vi "Temperature Controller Main.vi"() -> ()   [LabVIEW 2019, in "Controller.lvlib"]
uses:
  Controller.lvlib
  source code/LSL components/scripts/scripts manager/scripts manager.lvclass
  source code/LSL components/output terminal/Plain OT/PainOutputTerminal.lvclass
  D:/Pet Projects/LSL/source code/LSL components/output terminal/Base/Output Terminal.lvclass
  source code/LSL components/output terminal/Plain OT/PainOutputTerminal.lvclass/PainOutputTerminal.ctl
  source code/LSL components/variables/RT Variables/RT Variables.lvclass
  source code/LSL components/scripts/scripts manager/scripts manager.lvclass/scripts manager.ctl
  source code/LSL components/output terminal/Plain OT/properties/Write Output Terminal.vi
  source code/LSL components/scripts/scripts manager/properties/Write Scripts.vi
  customfunctions/ControllerData/ControllerData.lvclass
panel:
  out "Heater State":bool
  in  "Low Limit":dbl
  in  "High Limit":dbl
  out "CurrentTemperature":dbl(slide) scale=0.0..100.0
  out "Heater State Trend":i16(graph)
  out "Temperature Trend":T1(graph)
  in  "Script Run":bool
  in  "Script Editor":string
  out "Output Terminal":string
  # "Temperature Controller running on windows"
  # "Debug Console"
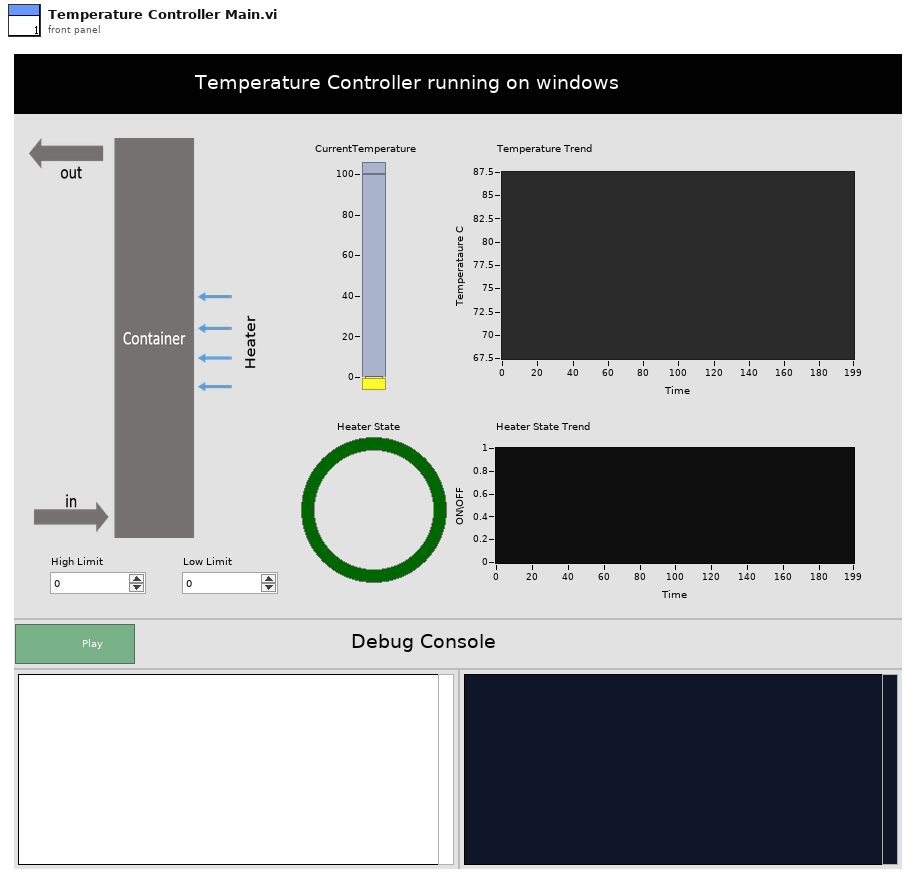
[diagram p1: front panel]
types:
  T1 = cluster{"Current Temp":dbl, "Low Set Point":dbl, "High Set Point":dbl}
  T2 = enum32{"invalid app kind", "Development System", "Run Time System", "Student Edition", "Embedded LabVIEW", "Evaluation", "Custom"}
  T3 = cluster{"Current Temp":dbl, "Low Set Point":dbl, "High Set Point":dbl}[]
  T4 = enum32{"Invalid", "Standard", "Closed", "Hidden", "Minimized", "Maximized"}
  T5 = cluster{"Core":cluster{"Current VI Reference":refnum<vi>, "Close Panel on Exit?":bool}, "High Set Point":dbl, "Low Set Point":dbl, "Current Temp":dbl, "Heater ON?":bool, "scripts manager":refnum<class "scripts manager.lvclass">, "Terminal":refnum<class "PainOutputTerminal.lvclass">, "appended path":path}
  T6 = cluster{"Current VI Reference":refnum<vi>, "Close Panel on Exit?":bool}
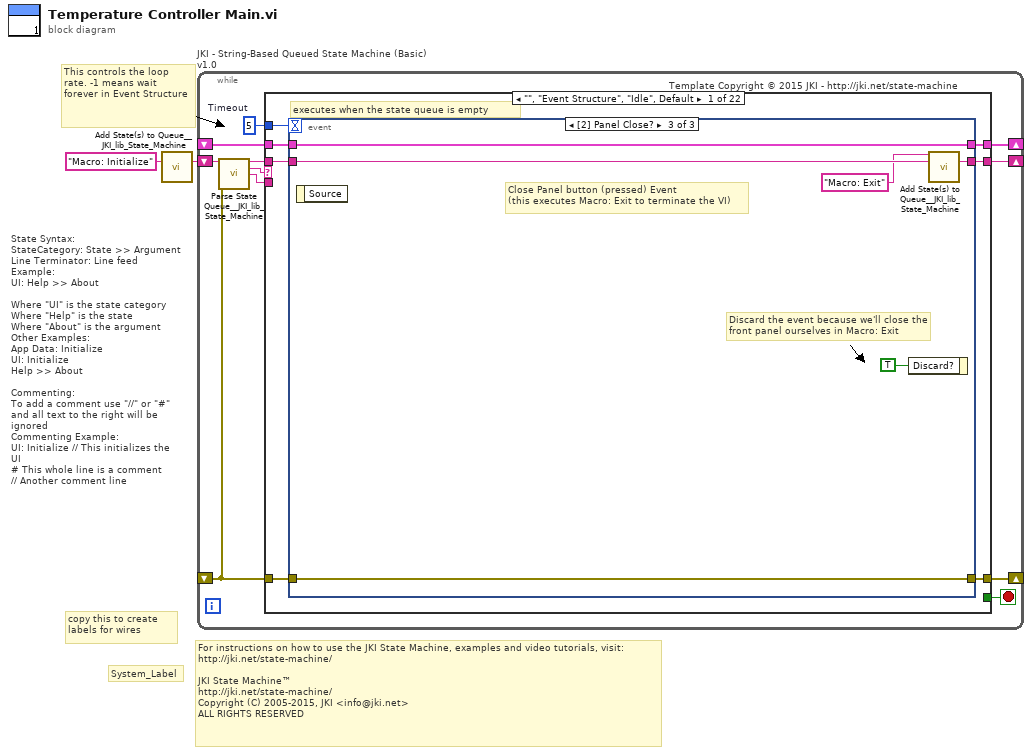
[diagram p0: block diagram]
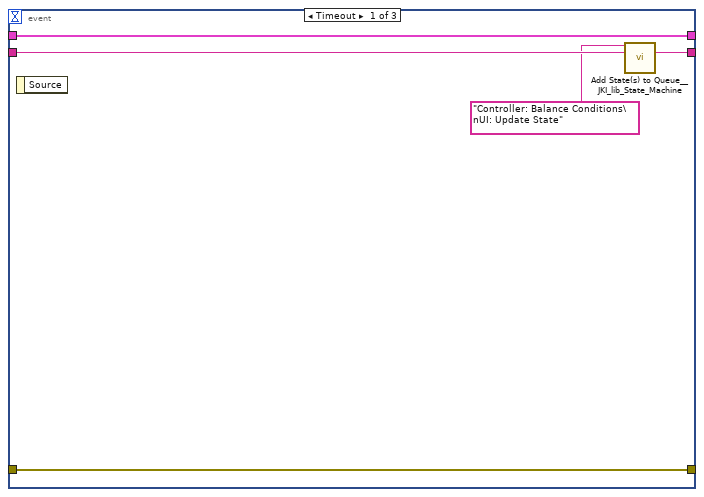
[diagram p2: hidden frame]
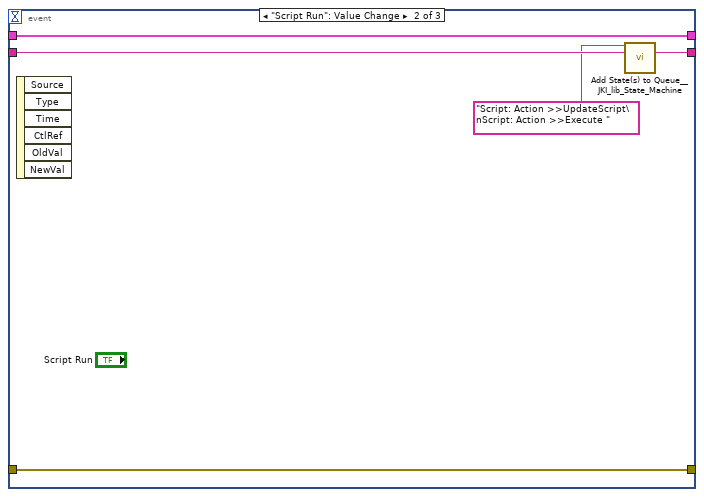
[diagram p3: hidden frame]
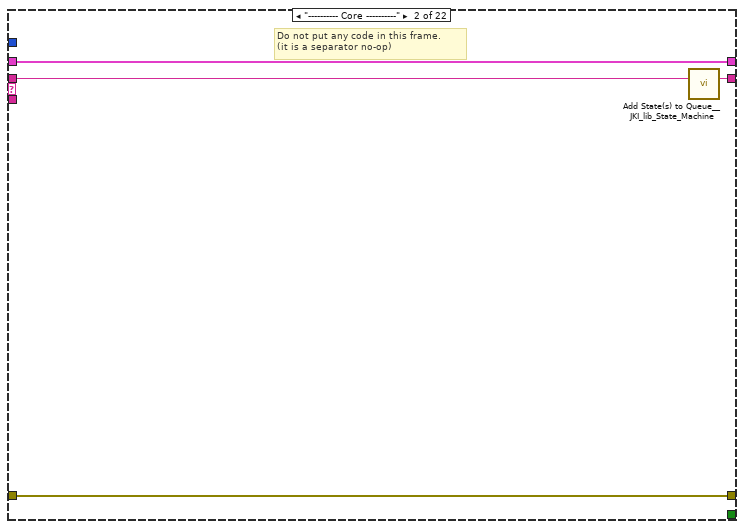
[diagram p4: hidden frame]
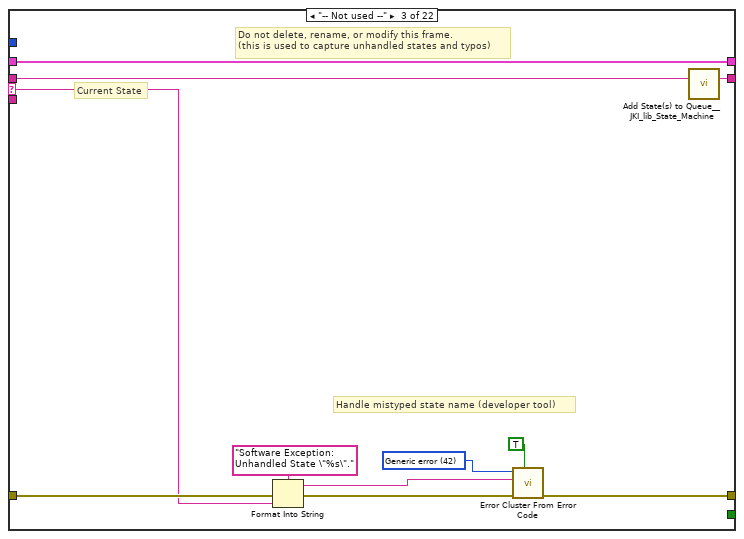
[diagram p5: hidden frame]
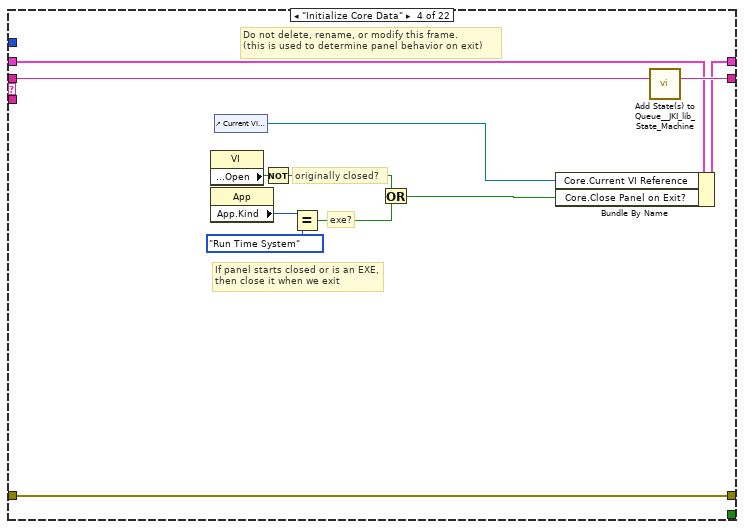
[diagram p6: hidden frame]
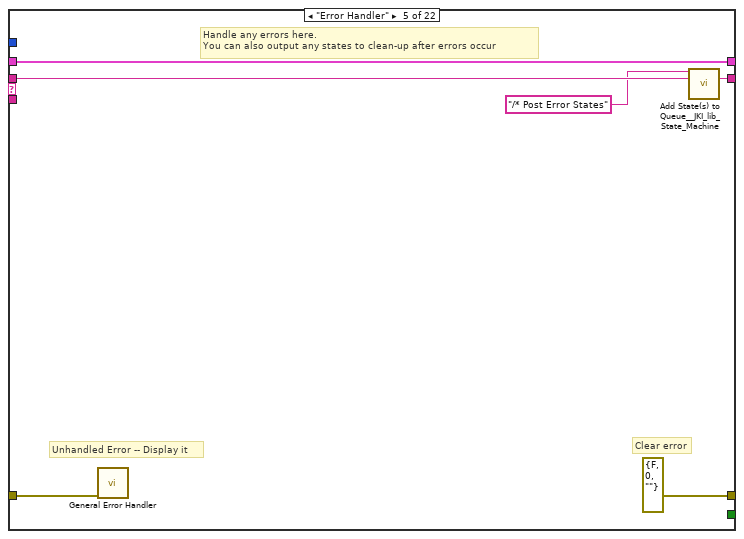
[diagram p7: hidden frame]
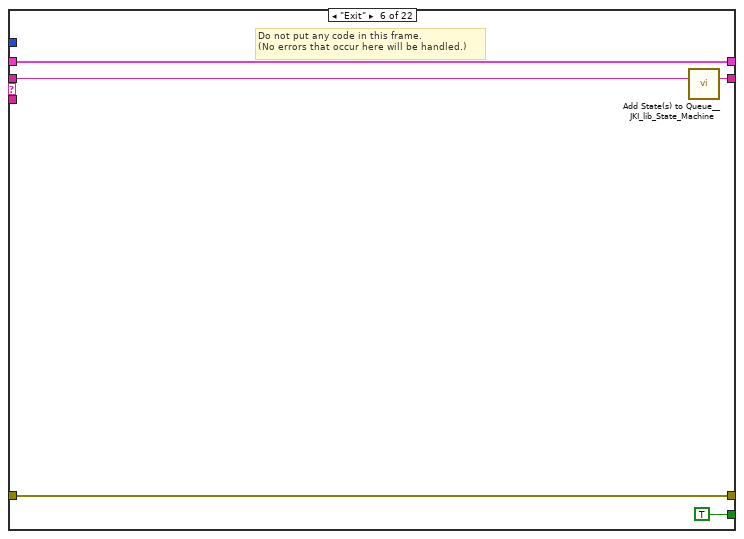
[diagram p8: hidden frame]
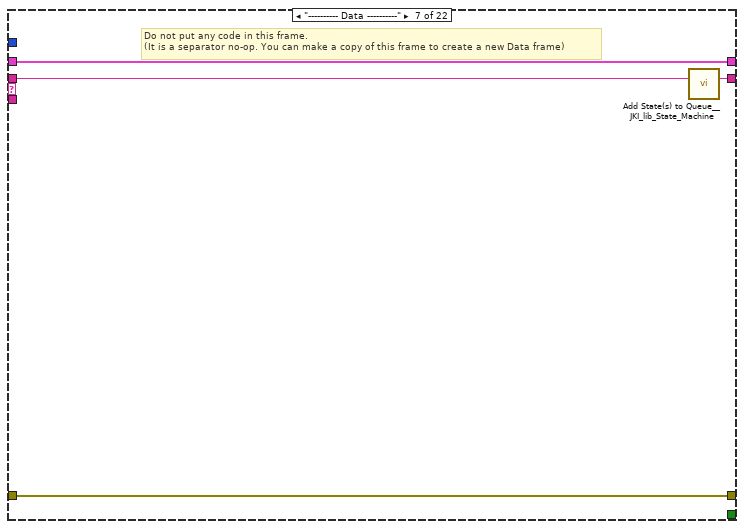
[diagram p9: hidden frame]
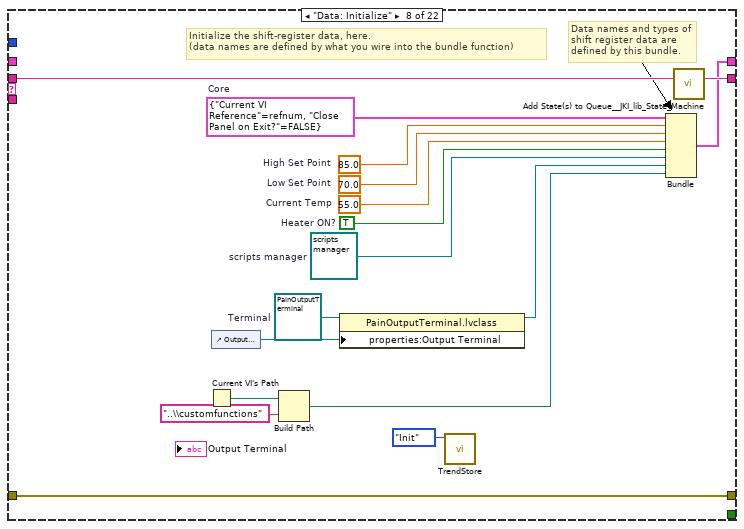
[diagram p10: hidden frame]
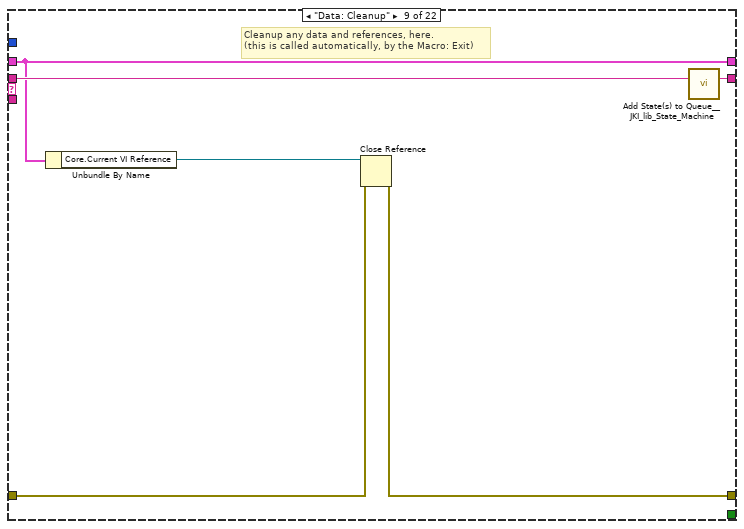
[diagram p11: hidden frame]
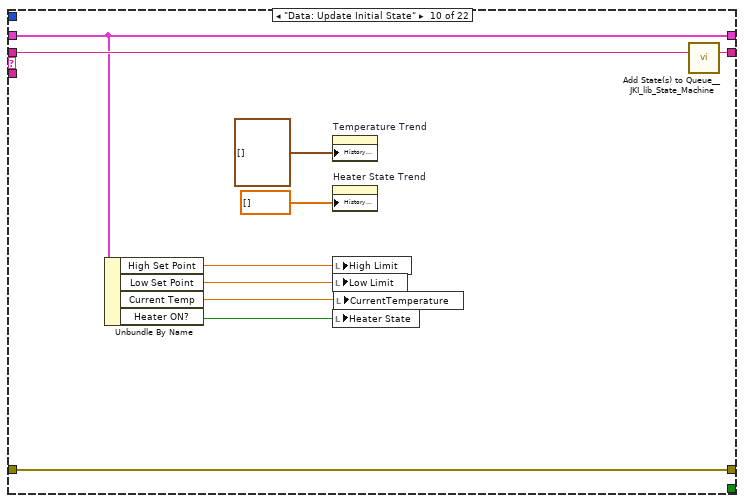
[diagram p12: hidden frame]
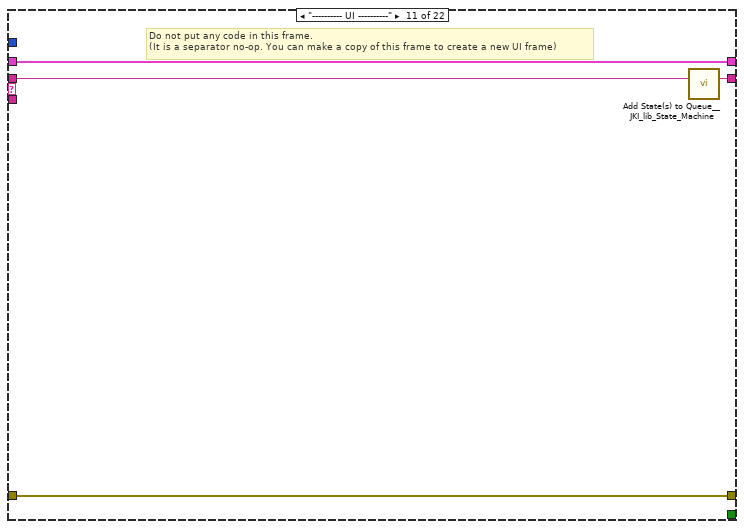
[diagram p13: hidden frame]
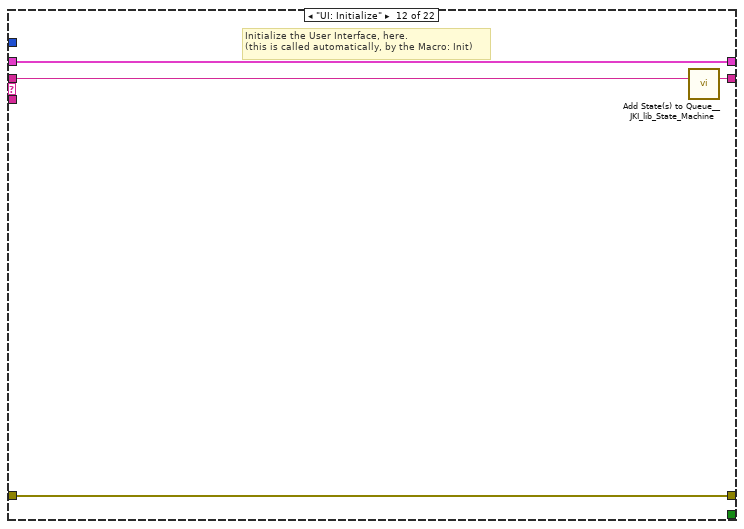
[diagram p14: hidden frame]
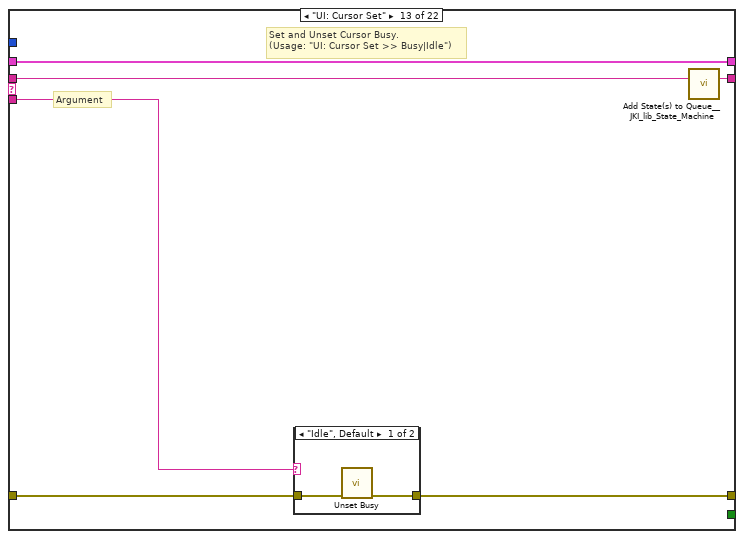
[diagram p15: hidden frame]
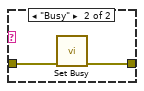
[diagram p16: hidden frame]
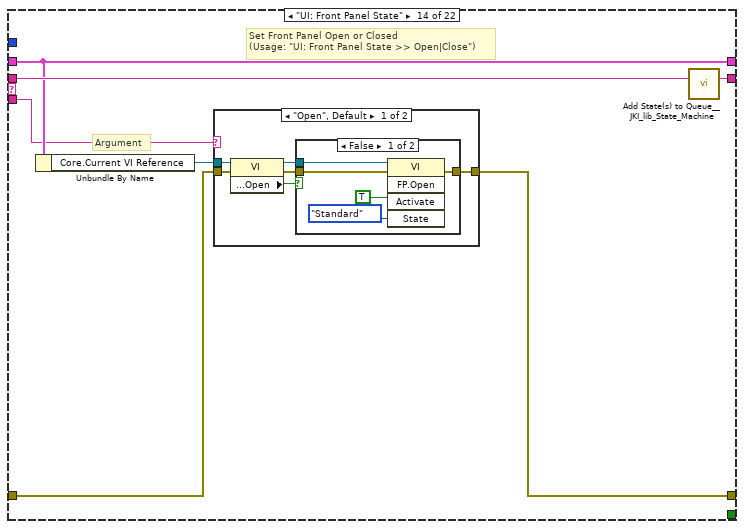
[diagram p17: hidden frame]
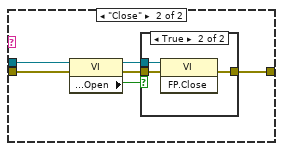
[diagram p19: hidden frame]
diagram:
  # "For instructions on how to use the JKI State Machine, examples and video tutorials, visit:\nhttp://jki.net/state-machine/\n\nJKI State Machine™\nhttp://jki.net/state-machine/\nCopyright (C) 2005-2015, JKI <info@jki.net>\nALL RIGHTS RESERVED"
  # "State Syntax:\nStateCategory: State >> Argument\nLine Terminator: Line feed\nExample:\nUI: Help >> About\n\nWhere \"UI\" is the state category\nWhere \"Help\" is the state\nWhere \"About\" is the argument\nOther Examples:\nApp Data: Initialize\nUI: Initialize\nHelp >> About\n\nCommenting:\nTo add a comment use \"//\" or \"#\" and all text to the right will be ignored\nCommenting Example:\nUI: Initialize // This initializes the UI\n# This whole line is a comment\n// Another comment line"
  # "copy this to create labels for wires"
  # "This controls the loop rate. -1 means wait forever in Event Structure"
  # "System_Label"
  n1 = call <vilib>:"Add State(s) to Queue__JKI_lib_State_Machine.vi"("State(s) in (\"\")"="Macro: Initialize") -> ("States Out"=w2:string)  [unwired: 14 in]
  n2 = while "JKI - String-Based Queued State Machine (Basic) v1.0" {
    shift-right: [w6] -> _
    shift-left: _ -> [w5]
    shift-right: [w9] -> _
    shift-left: _ -> [w3]
    shift-right: [w8] -> _
    shift-left: w2 -> [w10]
    stop <- w7 stop-if-true
    w4 = 5  # Timeout
    # "Template Copyright © 2015 JKI - http://jki.net/state-machine"
    n3 = call <vilib>:"Parse State Queue__JKI_lib_State_Machine.vi"("State Queue"=w10, "Error In (no error)"=w3) -> ("Remaining States"=w12:string, "Current State"=w13:string, "Arguments"=w11:string)  [unwired: 11 in]
    n4 = case shown="\"\", \"Event Structure\", \"Idle\", Default" w13 {
      selector: w13 -> [_ _ w41 _ _ _ _ _ _ _ _ _ _ _ _ _ _ _ _ _ _ _]
      tunnel: w12 -> [w20 w40 w45 w63 w69 w74 w78 w95 w101 w111 w115 w119 w125 w136 w167 w172 w177 w187 w191 w210 w212 w223]
      tunnel: w11 -> [_ _ _ _ _ _ _ _ _ _ _ _ w120 w130 _ _ _ _ _ _ _ w222]
      tunnel: w5 -> [w18 w37 w43 w54 w66 w72 w75 _ w96 w106 w112 w117 w123 w132 w165 w169 w174 w184 w188 w205 w213 w218]
      tunnel: [w17 w38 w47 w60 errorcluster {"status"=FALSE, "code"=0, "source"=""} ("error out") w71 w76 w92 w97 w109 w113 w116 w121 w133 w168 w170 w175 w185 w189 w208 w211 w216] -> w9
      tunnel: w3 -> [w16 w38 w46 w60 w65 w71 w76 w92 w98 w109 w113 w116 w122 w134 w168 w170 w175 w185 w189 w208 w211 w217]
      tunnel: [w19 w39 w44 w62 w68 w73 w77 w94 w100 w110 w114 w118 w124 w135 w166 w171 w176 w186 w190 w209 w212 w223] -> w8
      tunnel: [_ _ _ _ _ TRUE _ _ _ _ _ _ _ _ _ _ _ _ _ _ _ _] -> w7
      tunnel: [w15 w37 w43 w61 w66 w72 w75 w93 w96 w106 w112 w117 w123 w132 w165 w169 w174 w184 w188 w204 w213 w219] -> w6
      tunnel: w4 -> [w14 _ _ _ _ _ _ _ _ _ _ _ _ _ _ _ _ _ _ _ _ _]
      frame "", "Event Structure", "Idle", Default {
        # "executes when the state queue is empty"
        n5 = event shown="[2] Panel Close?" {
          selector: _ -> [_ _ _]
          dyn-events: _ -> [_ _ _]
          timeout: w14 -> [_ _ _]
          tunnel: w20 -> [w25 w30 w36]
          tunnel: [w24 w29 w35] -> w19
          tunnel: w18 -> [w22 w27 w33]
          tunnel: [w23 w28 w34] -> w17
          tunnel: w16 -> [w23 w28 w34]
          tunnel: [w22 w27 w33] -> w15
          event Timeout {
            n6 = event-data() -> ()  [unwired: 1 in, 1 out]
            n7 = call <vilib>:"Add State(s) to Queue__JKI_lib_State_Machine.vi"("State(s) in Front (\"\")"="Controller: Balance Conditions\nUI: Update State" ("State(s) in Front (\"\")"), "State(s) in (\"\")"=w25) -> ("States Out"=w24:string)  [unwired: 13 in]
          }
          event "Script Run": Value Change {
            n8 = event-data() -> ()  [unwired: 1 in, 6 out]
            n9 = call <vilib>:"Add State(s) to Queue__JKI_lib_State_Machine.vi"("State(s) in Front (\"\")"="Script: Action >>UpdateScript\nScript: Action >>Execute " ("State(s) in Front (\"\")"), "State(s) in (\"\")"=w30) -> ("States Out"=w29:string)  [unwired: 13 in]
          }
          event Panel Close? {
            # "Discard the event because we'll close the front panel ourselves in Macro: Exit"
            # "Close Panel button (pressed) Event\n(this executes Macro: Exit to terminate the VI)"
            n10 = event-data() -> ()  [unwired: 1 in, 1 out]
            n11 = event-data("Discard?"=TRUE) -> ()  [unwired: 1 in, 1 out]
            n12 = call <vilib>:"Add State(s) to Queue__JKI_lib_State_Machine.vi"("State(s) in Front (\"\")"="Macro: Exit", "State(s) in (\"\")"=w36) -> ("States Out"=w35:string)  [unwired: 13 in]
          }
        }
      }
      frame "---------- Core ----------" {
        # "Do not put any code in this frame.\n(it is a separator no-op)"
        n13 = call <vilib>:"Add State(s) to Queue__JKI_lib_State_Machine.vi"("State(s) in (\"\")"=w40) -> ("States Out"=w39:string)  [unwired: 14 in]
      }
      frame "-- Not used --" {
        w50 = 42 items=["No error", "Argument error", "Memory is full", "Out of zone", "End of file", "File already open", "Generic file I/O error", "File not found", "File permission error", "Disk is full", "Duplicate path", "Too many files open", "System feature not enabled", "Resource file not found", "Cannot add resource", "Resource not found", "Image not found", "Image memory error", "Pen does not exist", "Config type invalid", "Config token not found", "Config parse error", "Config memory error", "Bad external code format", "Bad external code offset", "External code not present", "Null window", "Destroy window error", "Null menu", "Print aborted", "Bad print record", "Print driver error", "Windows error during printing", "Memory error during printing", "Print dialog error", "Generic print error", "Invalid device refnum", "Device not found", "Device parameter error", "Device unit error", "Cannot open device", "Device call aborted", "Generic error", "Cancelled by user", "Object ID too low", "Object ID too high", "Object not in heap", "Unknown heap", "Unknown object (invalid DefProc)", "Unknown object (DefProc not in table)", "Message out of range", "Invalid (null) method", "Unknown message", "Manager call not supported", "Bad address", "Network operation in progress", "Network operation timed out", "Connection is busy", "Network attribute not supported", "Network error", "Address in use", "System out of memory", "Connection aborted", "Connection refused", "Not connected", "Already connected", "Connection closed", "Initialization error (interapplication manager)", "Bad occurrence", "Wait on unbound occurrence handler", "Occurrence queue overflow", "Datalog type conflict", "Unused", "Unrecognized type (interapplication manager)", "Memory corrupt", "Failed to make temporary DLL", "Old CIN version", "Drag socket not found", "Failed to load drop-object", "Failed to register OLE object", "Failed to release OLE object", "Format specifier type mismatch", "Unknown format specifier", "Too few format specifiers", "Too many format specifiers", "Scan failed", "Newer CIN version", "Error converting to variant", "Runtime menu error", "Password tampered", "Variant attribute not found", "Incompatible variant data type", "Event data is not available", "Event Store is not present", "Occurrence is not found", "Event Queue is not created", "Event info is not available", "Refnum passed is NULL", "Error retrieving Class GUID", "Error retrieving CoClass GUID", "Error retrieving TypeLib GUID.", "Bad built application magic bytes.", "Specific driver is different from the specific driver associated with the Logical Name.", "There is no session opened to the class driver.", "Max Error", "MAX - Error with config objects", "MAX - Error loading configuration", "MAX - Group not supported"]
        # "Current State"
        # "Do not delete, rename, or modify this frame.\n(this is used to capture unhandled states and typos)"
        # "Handle mistyped state name (developer tool)"
        n14 = Format Into String(format string="Software Exception: Unhandled State \"%s\"." ("message"), error in=w46, w41) -> (resulting string=w49:string, error out=w48:errorcluster)  [unwired: 1 in]
        n15 = call <vilib>:"Error Cluster From Error Code.vi"("show call chain? (False)"=TRUE, "error in (no error)"=w48, "error message (\"\")"=w49, "error code (0)"=w50) -> ("error out"=w47:errorcluster)  [unwired: 5 in]
        n16 = call <vilib>:"Add State(s) to Queue__JKI_lib_State_Machine.vi"("State(s) in (\"\")"=w45) -> ("States Out"=w44:string)  [unwired: 14 in]
      }
      frame "Initialize Core Data" {
        # "Do not delete, rename, or modify this frame.\n(this is used to determine panel behavior on exit)"
        # "originally closed?"
        # "exe?"
        # "If panel starts closed or is an EXE, then close it when we exit"
        n17 = property class="VI"() -> ("Front Panel.Open"=w59:bool)  [unwired: 2 in, 2 out]
        n18 = property class="App"() -> ("App.Kind"=w58:T2)  [unwired: 2 in, 2 out]
        n19 = control-ref of="Current VI Reference"() -> (w52:refnum<vi>)
        n20 = Not(x=w59) -> (.not. x?=w56:bool)
        n21 = Equal?(x=w58, y=T2."Run Time System" ("Application:Kind")) -> (x = y?=w55:bool)
        n22 = Or(x=w56, y=w55) -> (x .or. y?=w53:bool)
        n23 = Bundle By Name(cluster=w54, "Core.Current VI Reference"=w52, "Core.Close Panel on Exit?"=w53) -> (w61:T5)
        n24 = call <vilib>:"Add State(s) to Queue__JKI_lib_State_Machine.vi"("State(s) in (\"\")"=w63) -> ("States Out"=w62:string)  [unwired: 14 in]
      }
      frame "Error Handler" {
        # "Unhandled Error -- Display it"
        # "Handle any errors here.\nYou can also output any states to clean-up after errors occur"
        # "Clear error"
        n25 = call <vilib>:"General Error Handler.vi"("error in (no error)"=w65) -> ()  [unwired: 10 in, 5 out]
        n26 = call <vilib>:"Add State(s) to Queue__JKI_lib_State_Machine.vi"("State(s) in Front (\"\")"="/* Post Error States", "State(s) in (\"\")"=w69) -> ("States Out"=w68:string)  [unwired: 13 in]
      }
      frame "Exit" {
        # "Do not put any code in this frame.\n(No errors that occur here will be handled.)"
        n27 = call <vilib>:"Add State(s) to Queue__JKI_lib_State_Machine.vi"("State(s) in (\"\")"=w74) -> ("States Out"=w73:string)  [unwired: 14 in]
      }
      frame "---------- Data ----------" {
        # "Do not put any code in this frame.\n(It is a separator no-op. You can make a copy of this frame to create a new Data frame)"
        n28 = call <vilib>:"Add State(s) to Queue__JKI_lib_State_Machine.vi"("State(s) in (\"\")"=w78) -> ("States Out"=w77:string)  [unwired: 14 in]
      }
      frame "Data: Initialize" {
        w85 = refnum<class "PainOutputTerminal.lvclass"> refnum  # Terminal
        w86 = refnum<class "scripts manager.lvclass"> refnum  # scripts manager
        w87 = TRUE  # Heater ON?
        w88 = 55.0  # Current Temp
        w89 = 70.0  # Low Set Point
        w90 = 85.0  # High Set Point
        w91 = T6 {"Current VI Reference"=refnum, "Close Panel on Exit?"=FALSE}  # Core
        # "Data names and types of shift register data are defined by this bundle."
        # "Initialize the shift-register data, here.\n(data names are defined by what you wire into the bundle function)"
        n29 = Current VI's Path() -> (path=w82:path)
        n30 = control-ref of="Output Terminal"() -> (w84:refnum<vi>)
        n31 = Build Path(base path=w82, name or relative path="..\\customfunctions") -> (appended path=w80:path)
        n32 = property class="PainOutputTerminal.lvclass"(reference=w85, "properties:Output Terminal"=w84) -> (reference out=w83:refnum<class "PainOutputTerminal.lvclass">)  [unwired: 1 in, 1 out]
        n33 = call "TrendStore.vi"("Selector"=enum16{"Init", "Store", "Get"}."Init") -> ()  [unwired: 10 in, 1 out]
        n34 = Bundle("Core"=w91, "High Set Point"=w90, "Low Set Point"=w89, "Current Temp"=w88, "Heater ON?"=w87, "scripts manager"=w86, "Terminal"=w83, "appended path"=w80) -> (w93:T5)  [unwired: 1 in]
        n35 = call <vilib>:"Add State(s) to Queue__JKI_lib_State_Machine.vi"("State(s) in (\"\")"=w95) -> ("States Out"=w94:string)  [unwired: 14 in]
      }
      frame "Data: Cleanup" {
        # "Cleanup any data and references, here.\n(this is called automatically, by the Macro: Exit)"
        n36 = Unbundle By Name(w96) -> ("Core.Current VI Reference"=w99:refnum<vi>)
        n37 = Close Reference(reference=w99, error in (no error)=w98) -> (error out=w97:errorcluster)
        n38 = call <vilib>:"Add State(s) to Queue__JKI_lib_State_Machine.vi"("State(s) in (\"\")"=w101) -> ("States Out"=w100:string)  [unwired: 14 in]
      }
      frame "Data: Update Initial State" {
        n39 = Unbundle By Name(w106) -> ("High Set Point"=w105:dbl, "Low Set Point"=w104:dbl, "Current Temp"=w102:dbl, "Heater ON?"=w103:bool)
        n40 = property on="Temperature Trend" class="WFChart (strict)"("History Data"=T3 []) -> ()  [unwired: 2 in, 2 out]
        n41 = property on="Heater State Trend" class="WFChart (strict)"("History Data"=dbl[] []) -> ()  [unwired: 2 in, 2 out]
        n42 = local write "High Limit"(w105) -> ()
        n43 = local write "Low Limit"(w104) -> ()
        n44 = local write "Heater State"(w103) -> ()
        n45 = local write "CurrentTemperature"(w102) -> ()
        n46 = call <vilib>:"Add State(s) to Queue__JKI_lib_State_Machine.vi"("State(s) in (\"\")"=w111) -> ("States Out"=w110:string)  [unwired: 14 in]
      }
      frame "---------- UI ----------" {
        # "Do not put any code in this frame.\n(It is a separator no-op. You can make a copy of this frame to create a new UI frame)"
        n47 = call <vilib>:"Add State(s) to Queue__JKI_lib_State_Machine.vi"("State(s) in (\"\")"=w115) -> ("States Out"=w114:string)  [unwired: 14 in]
      }
      frame "UI: Initialize" {
        # "Initialize the User Interface, here.\n(this is called automatically, by the Macro: Init)"
        n48 = call <vilib>:"Add State(s) to Queue__JKI_lib_State_Machine.vi"("State(s) in (\"\")"=w119) -> ("States Out"=w118:string)  [unwired: 14 in]
      }
      frame "UI: Cursor Set" {
        # "Argument"
        # "Set and Unset Cursor Busy.\n(Usage: \"UI: Cursor Set >> Busy|Idle\")"
        n49 = case shown="\"Idle\", Default" w120 {
          tunnel: w122 -> [w127 w129]
          tunnel: [w126 w128] -> w121
          frame "Idle", Default {
            n50 = call <vilib>:"Unset Busy.vi"("error in (no error)"=w127) -> ("error out"=w126:errorcluster)  [unwired: 10 in]
          }
          frame "Busy" {
            n51 = call <vilib>:"Set Busy.vi"("error in (no error)"=w129) -> ("error out"=w128:errorcluster)  [unwired: 9 in, 1 out]
          }
        }
        n52 = call <vilib>:"Add State(s) to Queue__JKI_lib_State_Machine.vi"("State(s) in (\"\")"=w125) -> ("States Out"=w124:string)  [unwired: 14 in]
      }
      frame "UI: Front Panel State" {
        # "Argument"
        # "Set Front Panel Open or Closed\n(Usage: \"UI: Front Panel State >> Open|Close\")"
        n53 = Unbundle By Name(w132) -> ("Core.Current VI Reference"=w131:refnum<vi>)
        n54 = case shown="\"Open\", Default" w130 {
          tunnel: w134 -> [w140 w153]
          tunnel: [w142 w154] -> w133
          tunnel: w131 -> [w141 w151]
          frame "Open", Default {
            n55 = property class="VI"(reference=w141, error in=w140) -> (reference out=w138:refnum<vi>, error out=w139:errorcluster, "Front Panel.Open"=w137:bool)
            n56 = case shown="False" w137 {
              tunnel: [w145 w148] -> w142
              tunnel: w139 -> [w144 w148]
              tunnel: w138 -> [w143 _]
              frame False {
                n57 = invoke class="VI" method="FP.Open"(reference=w143, error in=w144, "Activate"=TRUE, "State"=T4."Standard") -> (error out=w145:errorcluster)  [unwired: 1 in, 4 out]
              }
              frame True {
              }
            }
          }
          frame "Close" {
            n58 = property class="VI"(reference=w151, error in=w153) -> (reference out=w150:refnum<vi>, error out=w152:errorcluster, "Front Panel.Open"=w149:bool)
            n59 = case shown="True" w149 {
              tunnel: [w155 w158] -> w154
              tunnel: w152 -> [w155 w157]
              tunnel: w150 -> [_ w156]
              frame False {
              }
              frame True {
                n60 = invoke class="VI" method="FP.Close"(reference=w156, error in=w157) -> (error out=w158:errorcluster)  [unwired: 1 in, 2 out]
              }
            }
          }
        }
        n61 = call <vilib>:"Add State(s) to Queue__JKI_lib_State_Machine.vi"("State(s) in (\"\")"=w136) -> ("States Out"=w135:string)  [unwired: 14 in]
      }
      frame "UI: Update State" {
        n62 = Unbundle By Name(w165) -> ("High Set Point"=w160:dbl, "Low Set Point"=w161:dbl, "Current Temp"=w162:dbl, "Heater ON?"=w163:bool)
        "CurrentTemperature" <- w162
        "Heater State" <- w163
        n63 = Boolean To (0,1)(Boolean=w163) -> (0, 1=→"Heater State Trend":i16)
        n64 = Bundle("Current Temp"=w162, "Low Set Point"=w161, "High Set Point"=w160) -> (→"Temperature Trend":T1)  [unwired: 1 in]
        n65 = call <vilib>:"Add State(s) to Queue__JKI_lib_State_Machine.vi"("State(s) in (\"\")"=w167) -> ("States Out"=w166:string)  [unwired: 14 in]
      }
      frame "---------- Macro ----------" {
        # "Do not put any code in this frame.\n(It is a separator no-op. You can make a copy of this frame to create a new Macro frame)"
        n66 = call <vilib>:"Add State(s) to Queue__JKI_lib_State_Machine.vi"("State(s) in (\"\")"=w172) -> ("States Out"=w171:string)  [unwired: 14 in]
      }
      frame "Macro: Initialize" {
        w173 = "Data: Initialize\nInitialize Core Data\nUI: Initialize\nUI: Front Panel State >> Open\nData: Update Initial State\nUI: Update State\n\nScript: Action >>Instantiate "  # Data: Initialize Initialize Core Data UI: Initialize UI: Front Panel State >> Open Data: Update Initial State UI: Update State  Script: Action >>Instantiate
        # "Initialization Macro\n(This is called once, when the VI starts)"
        n67 = call <vilib>:"Add State(s) to Queue__JKI_lib_State_Machine.vi"("State(s) in Front (\"\")"=w173, "State(s) in (\"\")"=w177) -> ("States Out"=w176:string)  [unwired: 13 in]
      }
      frame "Macro: Exit" {
        # "Exit Macro\n(This is called once, when the VI exits)"
        n68 = Unbundle By Name(w184) -> ("Core.Close Panel on Exit?"=w183:bool)
        n69 = Select(t="UI: Front Panel State >> Close", s=w183, f="") -> (s? t:f=w180:string)
        n70 = call <vilib>:"Add State(s) to Queue__JKI_lib_State_Machine.vi"("State(s) in (\"\")"=w180, "State(s) at Back (\"\")"="Script: Action >>Destroy \nData: Cleanup\nExit") -> ("States Out"=w178:string)  [unwired: 13 in]
        n71 = call <vilib>:"Add State(s) to Queue__JKI_lib_State_Machine.vi"("State(s) in Front (\"\")"=w178, "State(s) in (\"\")"=w187) -> ("States Out"=w186:string)  [unwired: 13 in]
      }
      frame "---------- Functions ----------" {
        # "Template Separator\n(You can make a copy of, or modify, this frame)"
        n72 = call <vilib>:"Add State(s) to Queue__JKI_lib_State_Machine.vi"("State(s) in (\"\")"=w191) -> ("States Out"=w190:string)  [unwired: 14 in]
      }
      frame "Controller: Balance Conditions" {
        # "Simulating a temperaure value to oscillate"
        n73 = Unbundle By Name(w205) -> ("Heater ON?"=w198:bool, "Current Temp"=w196:dbl)
        n74 = Max & Min(x="High Limit", y="Low Limit") -> (max(x,y)=w203:dbl, min(x,y)=w195:dbl)
        n75 = Less?(x=w196, y=w195) -> (x < y?=w194:bool)
        n76 = In Range and Coerce(upper limit=w203, x=w196, lower limit=w195) -> (In Range?=w199:bool)  [unwired: 1 out]
        n77 = Increment(x=w196) -> (x+1=w201:dbl)
        n78 = Decrement(x=w196) -> (x-1=w202:dbl)
        n79 = Select(t=w198, s=w199, f=w194) -> (s? t:f=w197:bool)
        n80 = Select(t=w201, s=w197, f=w202) -> (s? t:f=w193:dbl)
        n81 = Bundle By Name(cluster=w205, "High Set Point"=w203, "Low Set Point"=w195, "Heater ON?"=w197, "Current Temp"=w193) -> (w204:T5)
        n82 = Wait (ms)(milliseconds to wait=u32 300) -> ()  [unwired: 1 out]
        n83 = call "TrendStore.vi"("Temperature Value"=w193, "Selector"=enum16{"Init", "Store", "Get"}."Store") -> ()  [unwired: 9 in, 1 out]
        n84 = call <vilib>:"Add State(s) to Queue__JKI_lib_State_Machine.vi"("State(s) in (\"\")"=w210) -> ("States Out"=w209:string)  [unwired: 14 in]
      }
      frame "------------ Script--------------" {
      }
      frame "Script: Action" {
        n85 = Unbundle By Name(w218) -> ("appended path"=w214:path, "Terminal"=w215:refnum<class "PainOutputTerminal.lvclass">, "scripts manager"=w221:refnum<class "scripts manager.lvclass">)
        n86 = case shown="\"Execute\"" w222 {
          tunnel: w221 -> [_ w236 w241 w244]
          tunnel: [w229 w233 w237 refnum<class "scripts manager.lvclass"> refnum ("scripts manager out")] -> w220
          tunnel: w217 -> [w231 w235 w242 w246]
          tunnel: [w230 w232 w238 w245] -> w216
          tunnel: w215 -> [w227 _ _ _]
          tunnel: w214 -> [w225 _ _ _]
          frame "Instantiate", Default {
            n87 = Build Array(w225) -> (w224:path[])
            n88 = call-dynamic "Instantiate.vi"("scripts manager in"=refnum<class "scripts manager.lvclass"> refnum, "Output Terminal"=w227, "RT Variables"=refnum<class "RT Variables.lvclass"> refnum, "Function Directory[]"=w224, "error in (no error)"=w231) -> ("scripts manager out"=w229:refnum<class "scripts manager.lvclass">, "error out"=w230:errorcluster)  [unwired: 9 in]
          }
          frame "UpdateScript" {
            n89 = property class="scripts manager.lvclass"(reference=w236, error in=w235, "properties:Scripts"="Script Editor") -> (reference out=w233:refnum<class "scripts manager.lvclass">, error out=w232:errorcluster)
          }
          frame "Execute" {
            n90 = call-dynamic "Compile Script.vi"("scripts manager in"=w241, "error in (no error)"=w242) -> ("scripts manager out"=w239:refnum<class "scripts manager.lvclass">, "error out"=w240:errorcluster)  [unwired: 12 in]
            n91 = call-dynamic "Execute Script.vi"("scripts manager in"=w239, "error in (no error)"=w240) -> ("scripts manager out"=w237:refnum<class "scripts manager.lvclass">, "error out"=w238:errorcluster)  [unwired: 12 in]
          }
          frame "Destroy" {
            n92 = call-dynamic "Destroy.vi"("scripts manager in"=w244, "error in (no error)"=w246) -> ("error out"=w245:errorcluster)  [unwired: 12 in, 1 out]
          }
        }
        n93 = Bundle By Name(cluster=w218, "scripts manager"=w220) -> (w219:T5)
      }
    }
  }
